vi "Text as Encoded Path (LabVIEW String).vi"(6 "error in":errorcluster, 9 "Text":string) -> (1 "Encoded Path":T1, 4 "error out":errorcluster)   [LabVIEW 2020, in "G-Unicode.lvlib"]
doc: "Converts the input string or path to a raw UTF-8 encoded LabVIEW path. Valid inputs are a UTF-8 String class, UTF-8 Path class, LabVIEW string, or LabVIEW path."
uses:
  G-Unicode.lvlib
  Types/Encoded UTF-8 Path.ctl
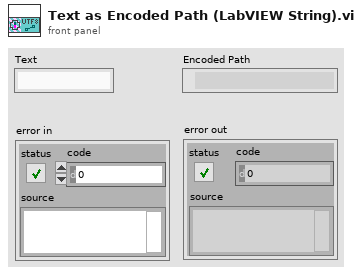
[diagram p1: front panel]
types:
  T1 = typedef "G-Unicode.lvlib/Encoded UTF-8 Path.ctl" = path
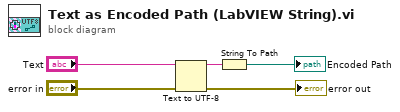
[diagram p0: block diagram]
diagram:
  n1 = Text to UTF-8(8:"error in", 11:"Text") -> (0:→"error out":errorcluster, 3:w1:string)  [unwired: 1 in]
  n2 = String To Path(string=w1) -> (path=→"Encoded Path":path)
